vi "Week_4_4.1_Ex-2.vi"() -> ()   [LabVIEW 2015]
panel:
  in  "Duty Cycle":dbl format="%#_13g"
  out "Waveform Graph":dynamicdata(graph)
  in  "Frequency":dbl format="%#_13g"
  in  "Peak value":dbl format="%#_13g"
  in  "Function":T1(ring)
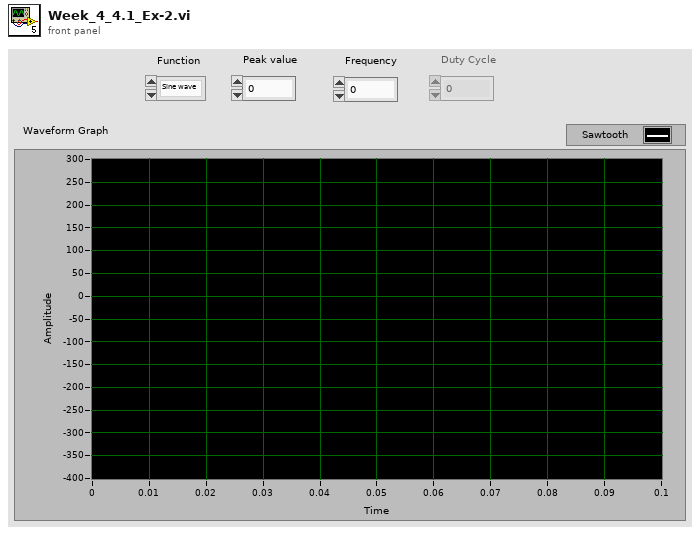
[diagram p1: front panel]
types:
  T1 = enum16{"Sine wave", "Sawtooth ", "Square", "Triangle", "Dc"}
  T2 = enum8{"Enabled", "Disabled", "Disabled and Grayed Out"}
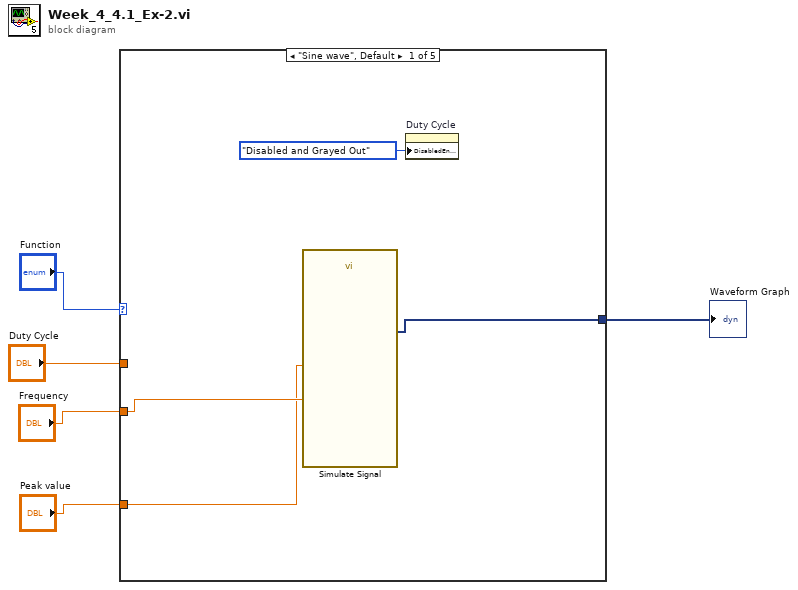
[diagram p0: block diagram]
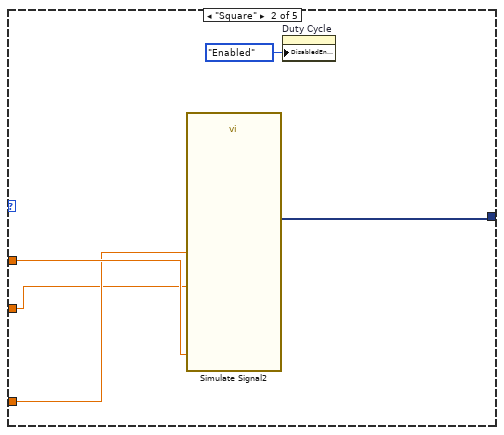
[diagram p2: hidden frame]
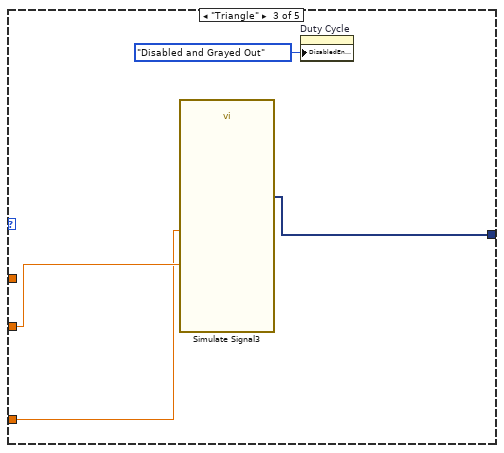
[diagram p3: hidden frame]
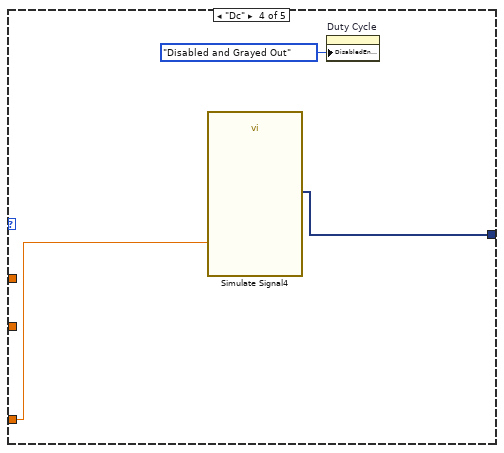
[diagram p4: hidden frame]
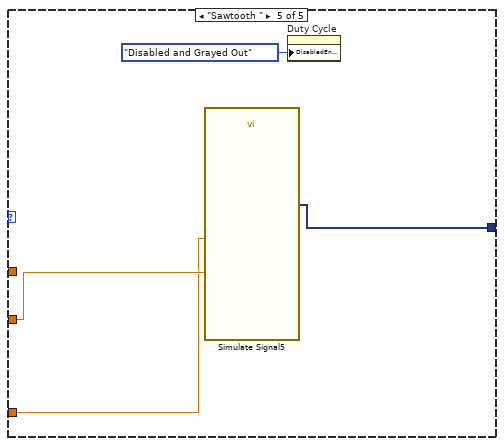
[diagram p5: hidden frame]
diagram:
  n1 = case shown="\"Sine wave\", Default" "Function" {
    tunnel: "Frequency" -> [w9 w11 w18 _ w25]
    tunnel: "Peak value" -> [w7 w12 w17 w21 w24]
    tunnel: [w8 w10 w16 w20 w22] -> w2
    tunnel: "Duty Cycle" -> [_ w14 _ _ _]
    frame "Sine wave", Default {
      n2 = call "Simulate Signal"("Frequency"=w9, "Amplitude"=w7) -> ("Sine"=w8:dynamicdata)  [unwired: 12 in, 1 out]
      n3 = property on="Duty Cycle" class="DigNum (strict)"("DisabledEnum"=T2."Disabled and Grayed Out" ("Disabled")) -> ()  [unwired: 2 in, 2 out]
    }
    frame "Square" {
      n4 = call "Simulate Signal2"("Duty Cycle (%)"=w14, "Frequency"=w11, "Amplitude"=w12) -> ("Square"=w10:dynamicdata)  [unwired: 11 in, 1 out]
      n5 = property on="Duty Cycle" class="DigNum (strict)"("DisabledEnum"=T2."Enabled" ("Disabled")) -> ()  [unwired: 2 in, 2 out]
    }
    frame "Triangle" {
      n6 = call "Simulate Signal3"("Frequency"=w18, "Amplitude"=w17) -> ("Triangle"=w16:dynamicdata)  [unwired: 12 in, 1 out]
      n7 = property on="Duty Cycle" class="DigNum (strict)"("DisabledEnum"=T2."Disabled and Grayed Out" ("Disabled")) -> ()  [unwired: 2 in, 2 out]
    }
    frame "Dc" {
      n8 = call "Simulate Signal4"("Offset"=w21) -> ("DC"=w20:dynamicdata)  [unwired: 13 in, 1 out]
      n9 = property on="Duty Cycle" class="DigNum (strict)"("DisabledEnum"=T2."Disabled and Grayed Out" ("Disabled")) -> ()  [unwired: 2 in, 2 out]
    }
    frame "Sawtooth " {
      n10 = call "Simulate Signal5"("Frequency"=w25, "Amplitude"=w24) -> ("Sawtooth"=w22:dynamicdata)  [unwired: 12 in, 1 out]
      n11 = property on="Duty Cycle" class="DigNum (strict)"("DisabledEnum"=T2."Disabled and Grayed Out" ("Disabled")) -> ()  [unwired: 2 in, 2 out]
    }
  }
  "Waveform Graph" <- w2
